vi "Main_03b.vi"() -> ()   [LabVIEW 2020]
uses:
  6bc75c88-cd30-4ad2-b351-994d74920a08.vi
  640cd243-7856-4436-86b5-240244b59ee9.vi
panel:
  out "array":string[](array[string])
  out "Array":i32[](array[numeric])
  out "sum":i32
  in  "Puzzle":string="DsPhSBQQQhqmBDhPDsFwjwsLjlRjlttvjvvtRb\nrNJMNNbrHrtjHLHjvwtg\nfNbNzZdrZnMnMPnQShFPDmnqFm\nQWVCFfQffgQCVZzVVpHsHJBqtpspJFRHqq\nmwDbmnnGNlNcwNDDNRbnNDlJTpBJBtJGtPTLsBGqTqqsqp\nMlSdnScRnnmmDjSdNSdCzvggWzrgzjvfvrgVzW\ngsMljbrjlZlWcWMJrWwTwbmwQbmmLDQQLhwL\nCdgpzdgpgnfThHfFRwhfRf\nSptgpSpnCNpVSGNPvPGSddcMWjMrjqBsJcWqMcBWcVlZ\nJcJLQQFWhQJPJpWcwjHvMQvnnlMvzBHd\ntCtGZrmVRmVGTVTtCfRTCHHNNvdNzmdMvMlNzvwdvw\nCTGGRftfSGtGTGDLbFchSgSWWWcM\nQcMFQrvrQbvtczbVbjbMzZzRpqmDDmqqnNzCDCDC\nSHHfPJssGLPSdHThLhHdRmqNmNssnNmNCNnpjmsn\nLhLJfTdLJwfgPTdfGccrtjcMrccwvcrrFr\njFLLLqDGjbtqLCChpMMhMBvpwMTmffpZ\nZnJHRncHHgnrsrZffTdMdMBfmMvfvR\nN..."
  in  "Example":string="vJrwpWtwJgWrhcsFMMfFFhFp\njqHRNqRjqzjGDLGLrsFMfFZSrLrFZsSL\nPmmdzqPrVvPwwTWBwg\nwMqvLMZHhHMvwLHjbvcjnnSBnvTQFn\nttgJtRGJQctTZtZT\nCrZsJsPPZsGzwwsLwLmpwMDw"
  # "2689"
  # "As you finish identifying the misplaced items, the Elves come to you with another issue.\n\nFor safety, the Elves are divided into groups of three. Every Elf carries a badge that identifies their group. For efficiency, within each group of three Elves, the badge is the only item type carried by all three Elves. That is, if a group's badge is item type B, then all three Elves will have item type B somewhere in their rucksack, and at most two of the Elves will be carrying any other item type.\n\nThe problem is that someone forgot to put this year's updated authenticity sticker on the badges. All of the badges need to be pulled out of the rucksacks so the new authenticity stickers can be attached.\n\nAdditionally, nobody wrote down which item type corresponds to each group's badges. The only way to tell which item type is the right one is by finding the one item type that is common between all three Elves in each group.\n\nEvery set of three lines in your list corresponds to a single group, but each group can have a different badge item type. So, in the above example, the first group's rucksacks are the first three lines:\n\nvJrwpWtwJgWrhcsFMMfFFhFp\njqHRNqRjqzjGDLGLrsFMfFZSrLrFZsSL\nPmmdzqPrVvPwwTWBwg\nAnd the second group's rucksacks are the next three lines:\n\nwMqvLMZHhHMvwLHjbvcjnnSBnvTQFn\nttgJtRGJQctTZtZT\nCrZsJsPPZsGzwwsLwLmpwMDw\nIn the first group, the only item type that appears in all three rucksacks is lowercase r; this must be their badges. In the second group, their badge item type must be Z.\n\nPriorities for these items must still be found to organize the sticker attachment efforts: here, they are 18 (r) for the first group and 52 (Z) for the second group. The sum of these is 70.\n\nFind the item type that corresponds to the badges of each three-Elf group. What is the sum of the priorities of those item types?"
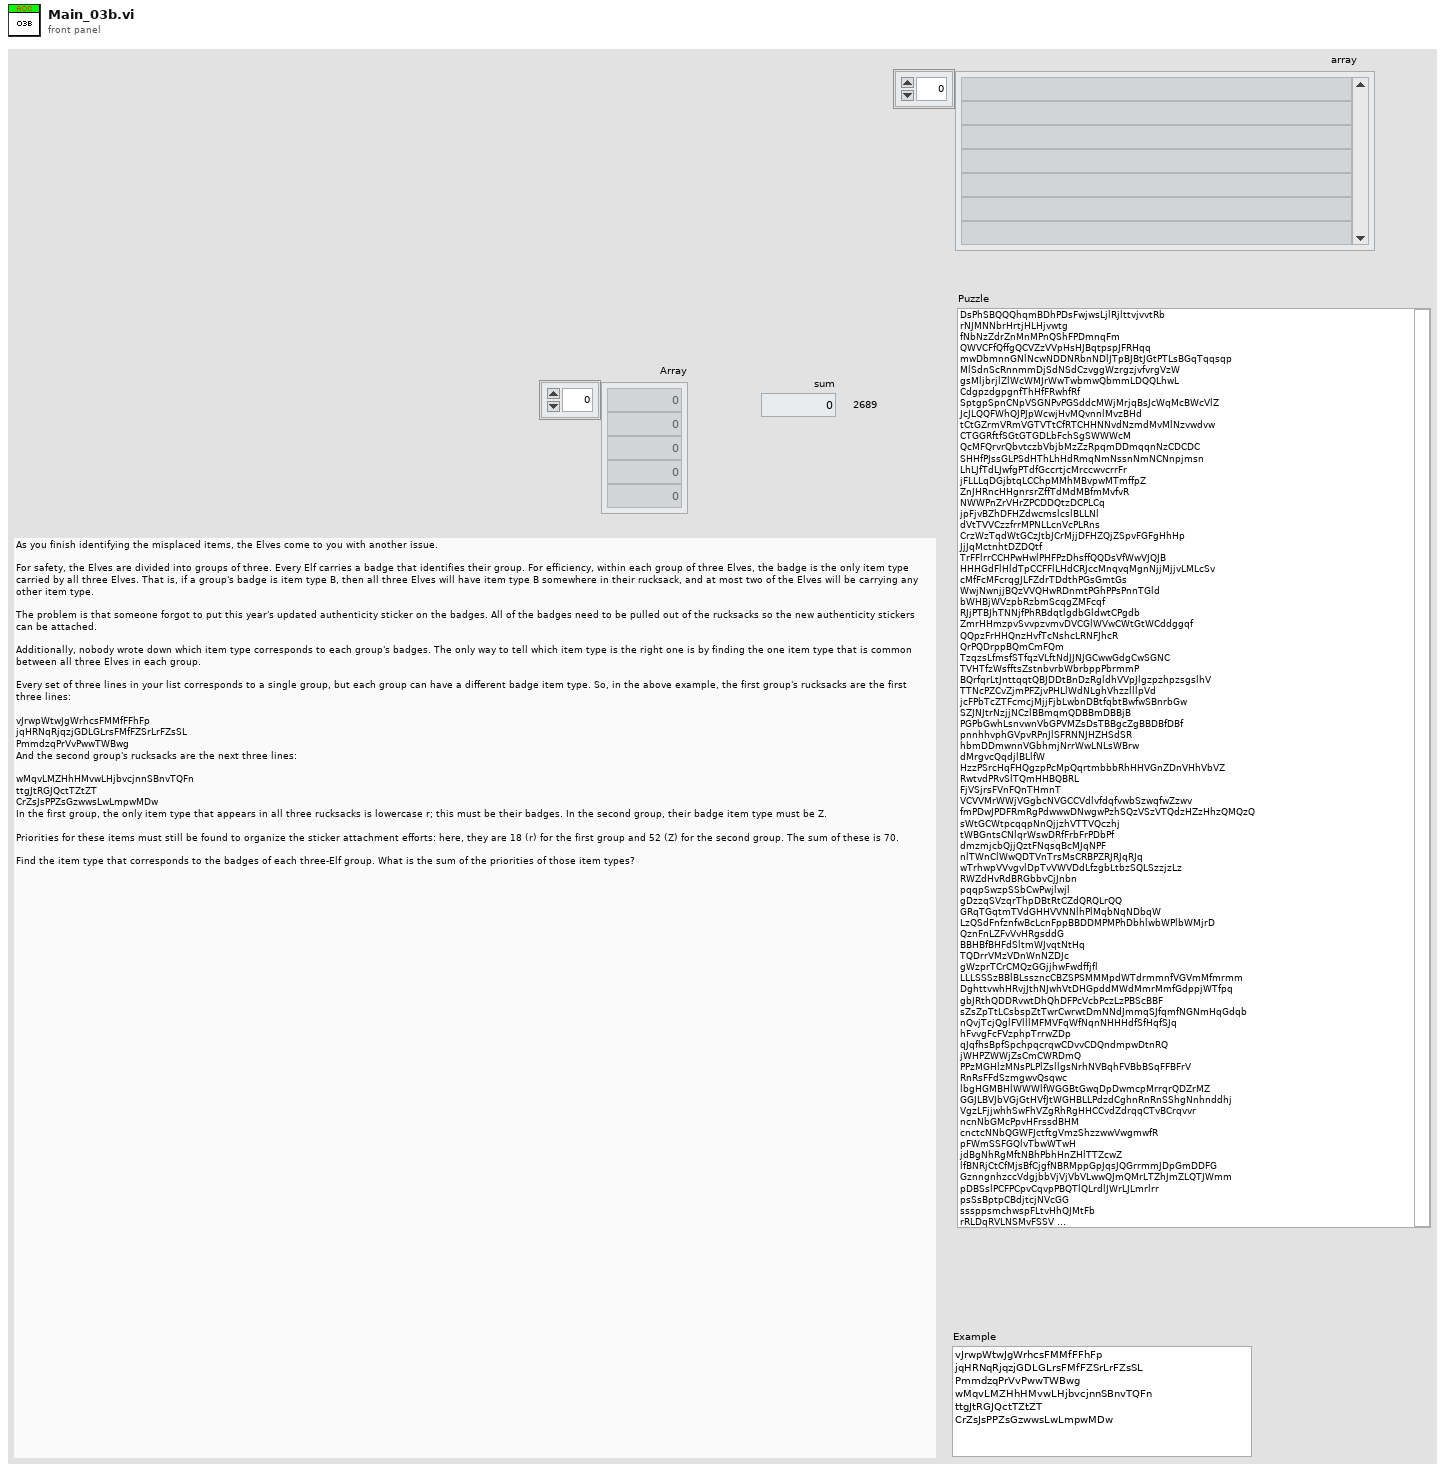
[diagram p1: front panel]
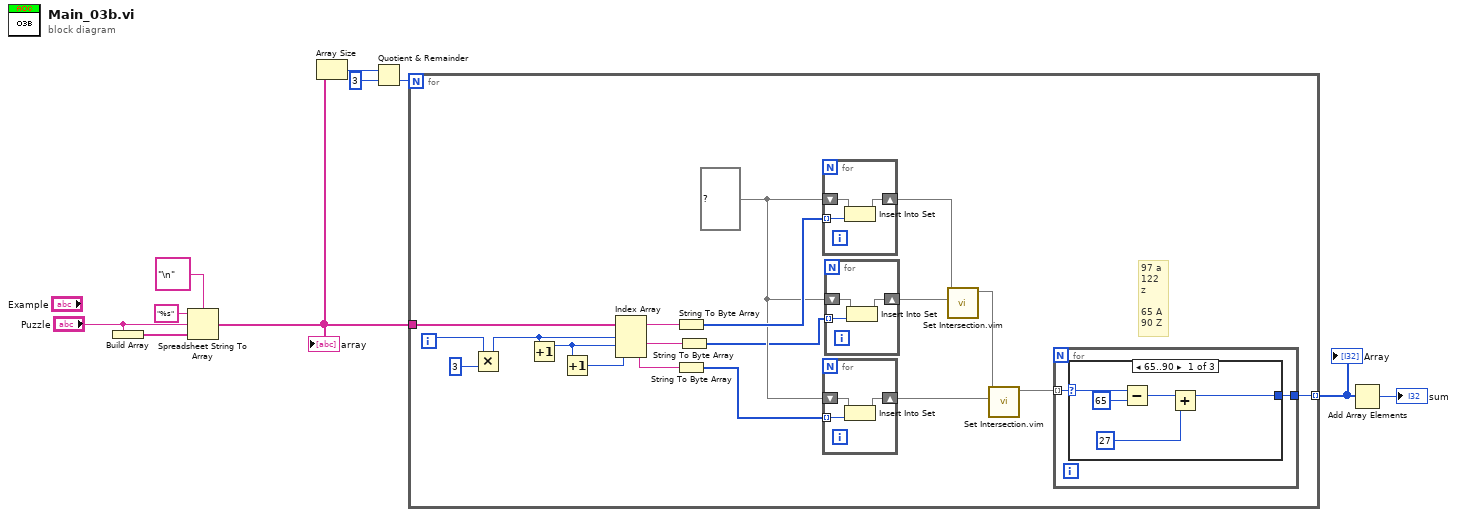
[diagram p0: block diagram]
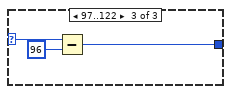
[diagram p3: hidden frame]
diagram:
  n1 = Build Array("Puzzle") -> (w10:string[])
  n2 = Spreadsheet String To Array(delimiter (Tab)="\n", format string="%s", spreadsheet string="Puzzle", array type (2D Dbl)=w10) -> (array=w5:string[])
  "array" <- w5
  n3 = Array Size(array=w5) -> (size(s)=w4:i32)
  n4 = Quotient & Remainder(x=w4, y=3) -> (floor(x/y)=w2:i32)  [unwired: 1 out]
  n5 = for {
    N: w2 -> [_]
    tunnel: [w29] -> w7 mode=indexing
    tunnel: w5 -> [w28]
    i -> [w21]
    w16 = set{u8} {} ("set")
    # "97 a\n122 z\n\n65 A\n90 Z"
    n6 = Multiply(x=w21, y=3) -> (x*y=w20:i32)
    n7 = Increment(x=w20) -> (x+1=w26:i32)
    n8 = Increment(x=w26) -> (x+1=w25:i32)
    n9 = Index Array(array=w28, index #1=w20, index #2=w26, index #3=w25) -> (element #1=w27:string, element #2=w24:string, element #3=w23:string)
    n10 = String To Byte Array(string=w27) -> (unsigned byte array=w19:u8[])
    n11 = String To Byte Array(string=w23) -> (unsigned byte array=w14:u8[])
    n12 = String To Byte Array(string=w24) -> (unsigned byte array=w15:u8[])
    n13 = for {
      tunnel: w19 -> [w37] mode=indexing
      shift-right: [w36] -> w13
      shift-left: w16 -> [w38]
      n14 = Insert Into Set(10:w37, 11:w38) -> (3:w36:set{u8})  [unwired: 1 out]
    }
    n15 = for {
      tunnel: w14 -> [w31] mode=indexing
      shift-right: [w30] -> w11
      shift-left: w16 -> [w32]
      n16 = Insert Into Set(10:w31, 11:w32) -> (3:w30:set{u8})  [unwired: 1 out]
    }
    n17 = for {
      tunnel: w15 -> [w34] mode=indexing
      shift-right: [w33] -> w12
      shift-left: w16 -> [w35]
      n18 = Insert Into Set(10:w34, 11:w35) -> (3:w33:set{u8})  [unwired: 1 out]
    }
    n19 = call "Set Intersection.vim"("set 2"=w12, "set 1"=w13) -> ("intersection"=w18:set{u8})  [unwired: 9 in]
    n20 = call "Set Intersection.vim"("set 2"=w11, "set 1"=w18) -> ("intersection"=w17:set{u8})  [unwired: 9 in]
    n21 = for {
      tunnel: [w40] -> w29
      tunnel: w17 -> [w39] mode=indexing
      n22 = case shown="65..90" w39 {
        selector: w39 -> [w45 w46 w49]
        tunnel: [w43 w46 w47] -> w40
        frame 65..90 {
          n23 = Subtract(x=w45, y=u8 65) -> (x-y=w44:u8)
          n24 = Add(x=w44, y=27) -> (x+y=w43:i32)
        }
        frame Default {
        }
        frame 97..122 {
          n25 = Subtract(x=w49, y=u8 96) -> (x-y=w47:u8)
        }
      }
    }
  }
  "Array" <- w7
  n26 = Add Array Elements(numeric array=w7) -> (sum=→"sum":i32)
